vi "test Cluster and Waveform Packing.vi"(8 "error in (no error)":errorcluster, 11 "TestCase in":refnum<class "Data Structure Tests.lvclass">) -> (0 "error out":errorcluster, 3 "TestCase out":refnum<class "Data Structure Tests.lvclass">)   [LabVIEW 2024, in "Data Structure Tests.lvclass"]
uses:
  Data Structure Tests.lvclass
  <vilib>/Utility/file.llb/Application Directory.vi
  <vilib>/Utility/libraryn.llb/Check if File or Folder Exists.vi
  Data Structure Tests.lvclass/Data Structure Tests.ctl
  <vilib>/addons/_JKI Toolkits/VI Tester/TestCase.llb/TestCase.lvclass
  C:/Program Files/National Instruments/LabVIEW 2024/vi.lib/addons/_JKI Toolkits/VI Tester/TestCase.llb/TestCase.lvclass
  C:/Users/JamesMcNally/Documents/WiresmithProjects/OpenSource/Rust-LabVIEW-Interop/labview-test-project/Data Structure Tests/Data Structure Tests.lvclass
panel:
  out "three":u32 format="%.0x"
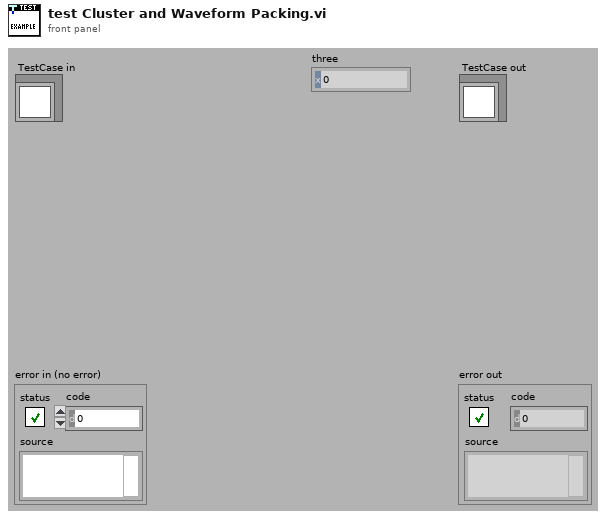
[diagram p1: front panel]
types:
  T1 = cluster{"one":u8, "two":u16, "waveform":waveform(dbl), "three":u32}
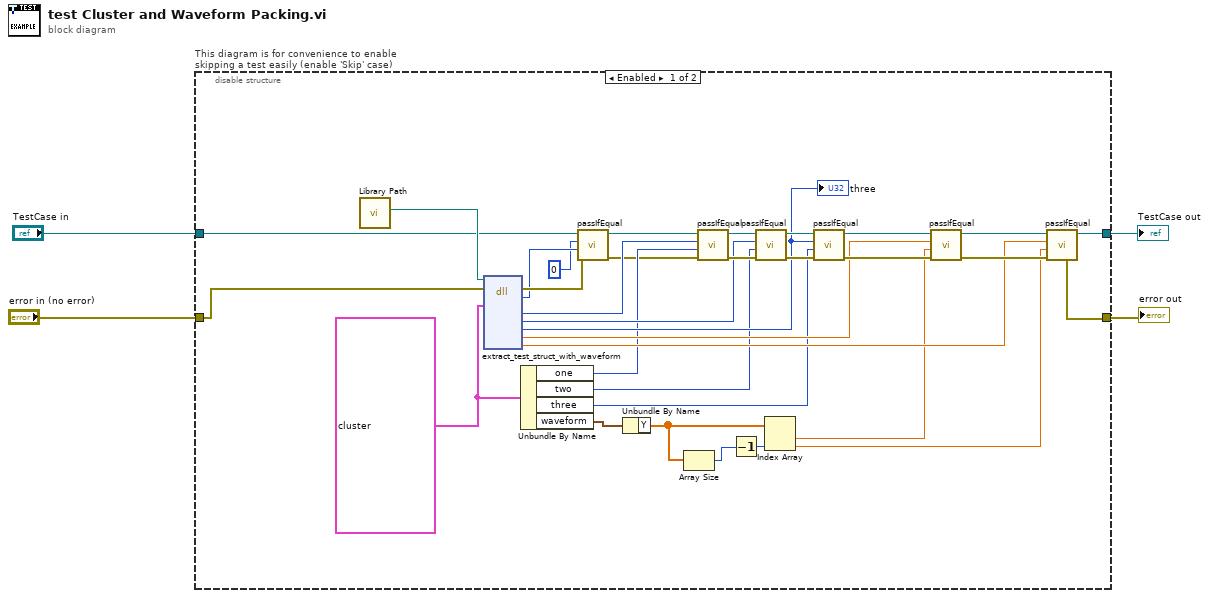
[diagram p0: block diagram]
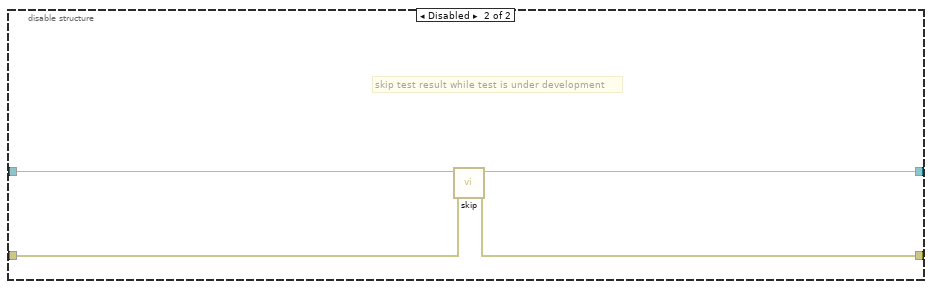
[diagram p2: hidden frame]
diagram:
  n1 = disable-structure "This diagram is for convenience to enable skipping a test easily (enable 'Skip' case)" shown="Enabled" {
    disable-tunnel: "TestCase in" -> [w8 w41]
    disable-tunnel: [w26 w39] -> w1
    disable-tunnel: [w28 w40] -> w3
    disable-tunnel: "error in (no error)" -> [w36 w38]
    frame Enabled {
      w20 = T1 {"one"=5, "two"=1024, "waveform"={"t0"=timestamp(3759079179.562472 s since 1904-01-01), "dt"=1.0, "Y"=[1.0, 2.0, 3.0]}, "three"=4096}
      n2 = call "Library Path.vi"() -> ("Library Path"=w10:path)  [unwired: 11 in]
      n3 = dll-call lib="C:/Users/JamesMcNally/Documents/RustInterop/Rust-LabVIEW-Interop/target/debug/labview_test_library.dll" fn="extract_test_struct_with_waveform"(path in=w10, error in=w36, "struct"=w20) -> (error out=w35:errorcluster, "error"=w6:i32, "one"=w25:u8, "two"=w24:u16, "three"=w23:u32, "wv_first"=w22:dbl, "wv_last"=w21:dbl)  [unwired: 7 in, 1 out]
      "three" <- w23
      n4 = Unbundle By Name(w20) -> ("one"=w19:u8, "two"=w18:u16, "three"=w17:u32, "waveform"=w16:waveform(dbl))
      n5 = call-dynamic "passIfEqual.vi"("error in (no error)"=w35, "y"=w6, "x"=0 ("error"), "TestCase in"=w8) -> ("error out"=w9:errorcluster, "TestCase out"=w7:refnum<class "Data Structure Tests.lvclass">)  [unwired: 6 in]
      n6 = Unbundle By Name(w16) -> ("Y"=w14:dbl[])
      n7 = Array Size(array=w14) -> (size(s)=w13:i32)
      n8 = call-dynamic "passIfEqual.vi"("error in (no error)"=w9, "y"=w19, "x"=w25, "TestCase in"=w7) -> ("error out"=w37:errorcluster, "TestCase out"=w30:refnum<class "Data Structure Tests.lvclass">)  [unwired: 6 in]
      n9 = Decrement(x=w13) -> (x-1=w12:i32)
      n10 = call-dynamic "passIfEqual.vi"("error in (no error)"=w37, "y"=w18, "x"=w24, "TestCase in"=w30) -> ("error out"=w31:errorcluster, "TestCase out"=w29:refnum<class "Data Structure Tests.lvclass">)  [unwired: 6 in]
      n11 = Index Array(array=w14, index #2=w12) -> (element #1=w15:dbl, element #2=w11:dbl)  [unwired: 1 in]
      n12 = call-dynamic "passIfEqual.vi"("error in (no error)"=w31, "y"=w17, "x"=w23, "TestCase in"=w29) -> ("error out"=w33:errorcluster, "TestCase out"=w32:refnum<class "Data Structure Tests.lvclass">)  [unwired: 6 in]
      n13 = call-dynamic "passIfEqual.vi"("error in (no error)"=w33, "y"=w15, "x"=w22, "TestCase in"=w32) -> ("error out"=w34:errorcluster, "TestCase out"=w27:refnum<class "Data Structure Tests.lvclass">)  [unwired: 6 in]
      n14 = call-dynamic "passIfEqual.vi"("error in (no error)"=w34, "y"=w11, "x"=w21, "TestCase in"=w27) -> ("error out"=w28:errorcluster, "TestCase out"=w26:refnum<class "Data Structure Tests.lvclass">)  [unwired: 6 in]
    }
    frame Disabled {
      # "skip test result while test is under development"
      n15 = call <vilib>:"skip.vi"("error in (no error)"=w38, "TestCase in"=w41) -> ("error out"=w40:errorcluster, "TestCase out"=w39:refnum<class "Data Structure Tests.lvclass">)  [unwired: 8 in]
    }
  }
  "error out" <- w3
  "TestCase out" <- w1
